vi "Actor Core.vi"(8 "error in":errorcluster, 11 "Measurement Señal Actualizable in":refnum<class "Measurement Señal Actualizable.lvclass">) -> (0 "error out":errorcluster, 3 "Actor out":refnum<class "Actor.lvclass">)   [LabVIEW 2020, in "Measurement Señal Actualizable.lvlib" / "Measurement Señal Actualizable.lvclass"]
doc: "(<B>Filename</B>: Actor Framework.lvlib:Actor.lvclass:Actor Core.vi)\n\nReceives messages to the actor, reacts to them, and initiates any error handling that may shut the actor down.\n\nDescendant classes may override this VI to append parallel tasks for the actor to complete while it handles messages. Overrides use the Call Parent Class Method node."
uses:
  C:/Program Files (x86)/National Instruments/LabVIEW 2020/vi.lib/ActorFramework/Actor/Actor.lvclass
  <vilib>/ActorFramework/Actor/Actor.lvclass
  <vilib>/ActorFramework/Actor/Actor.lvclass/Actor.ctl
  <vilib>/ActorFramework/Message Enqueuer/Message Enqueuer.lvclass/Message Enqueuer.ctl
  <vilib>/ActorFramework/Message Enqueuer/Enqueue.vi
  C:/Program Files (x86)/National Instruments/LabVIEW 2020/vi.lib/ActorFramework/Message/Message.lvclass
  <vilib>/ActorFramework/Message Priority Queue/Priority Enqueue.vi
  <vilib>/measure/NI_MABase.lvlib
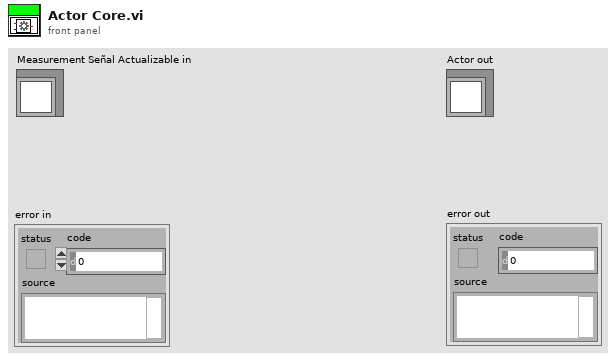
[diagram p1: front panel]
types:
  T1 = cluster{"frecuencia":dbl, "Amplitud":dbl, "Tipo de señal":enum16{"Sine Wave", "Triangle Wave", "Square Wave", "Sawtooth Wave"}}
  T2 = cluster{"Start/stop HL Event":refnum<user-event>, "Exit Event":refnum<user-event>, "Parametros Graph event":refnum<user-event>}
  T3 = enum16{"Sine Wave", "Triangle Wave", "Square Wave", "Sawtooth Wave"}
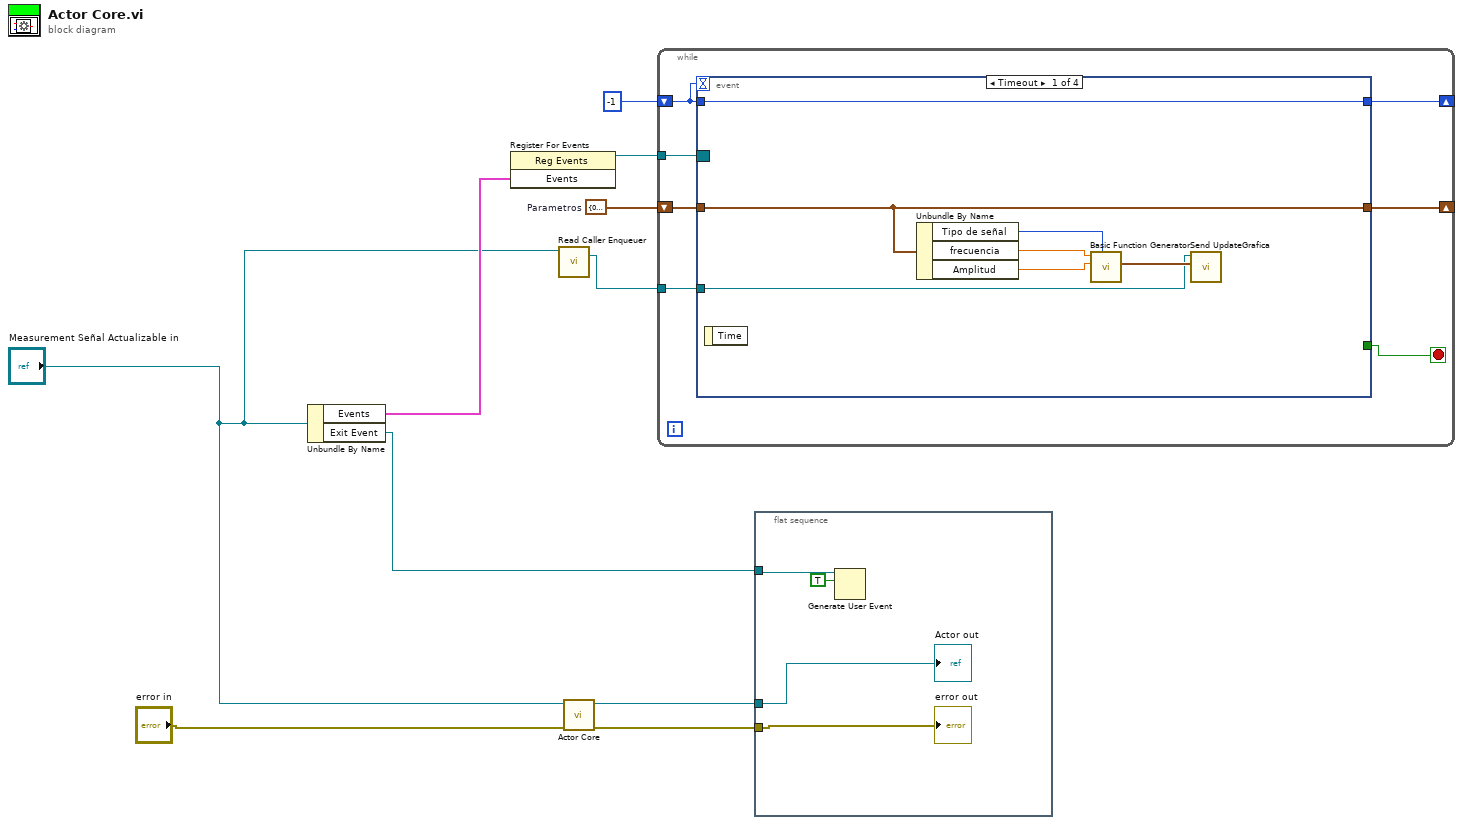
[diagram p0: block diagram]
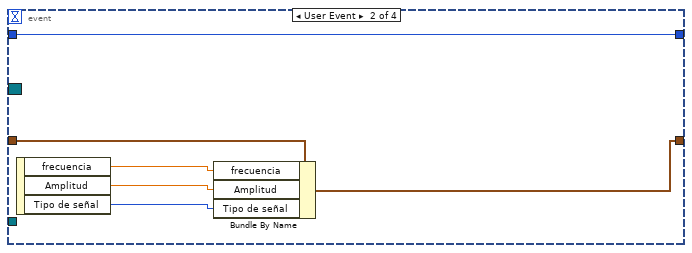
[diagram p2: hidden frame]
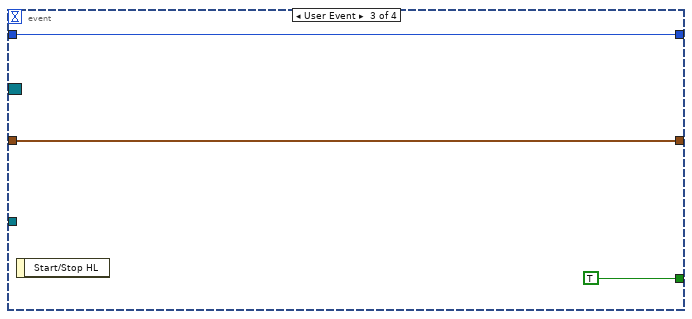
[diagram p3: hidden frame]
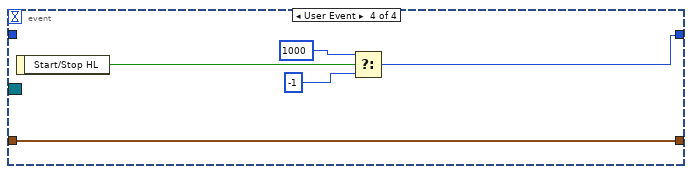
[diagram p4: hidden frame]
diagram:
  w2 = T1 {"frecuencia"=0.0, "Amplitud"=0.0, "Tipo de señal"=enum."Sine Wave"}  # Parametros
  n1 = Unbundle By Name("Measurement Señal Actualizable in") -> ("Events"=w6:T2, "Exit Event"=w7:refnum<user-event>)
  n2 = register-events(w6) -> (reference out=w4:refnum<event-registration>)  [unwired: 2 in, 1 out]
  n3 = call <vilib>:"Read Caller Enqueuer.vi"("Actor"="Measurement Señal Actualizable in") -> ("Caller Enqueuer"=w1:refnum<class "Message Enqueuer.lvclass">)  [unwired: 10 in]
  n4 = call-parent "Actor Core.vi"("error in"="error in", "Actor in"="Measurement Señal Actualizable in") -> ("error out"=w10:errorcluster, "Actor out"=w9:refnum<class "Actor.lvclass">)  [unwired: 8 in]
  n5 = while {
    tunnel: w4 -> [w17]
    shift-right: [w16] -> _
    shift-left: -1 -> [w15]
    shift-right: [w13] -> _
    shift-left: w2 -> [w14]
    tunnel: w1 -> [w12]
    stop <- w11 stop-if-true
    n6 = event shown="[0] Timeout" {
      selector: w17 -> [_ _ _ _]
      dyn-events: _ -> [_ _ _ _]
      timeout: w15 -> [_ _ _ _]
      tunnel: w15 -> [w24 w25 w33 _]
      tunnel: [w24 w25 w33 w34] -> w16
      tunnel: w14 -> [w23 w30 w32 w38]
      tunnel: [w23 w29 w32 w38] -> w13
      tunnel: w12 -> [w18 _ _ _]
      tunnel: [_ _ TRUE _] -> w11
      event Timeout {
        n7 = event-data() -> ()  [unwired: 1 in, 1 out]
        n8 = Unbundle By Name(w23) -> ("Tipo de señal"=w20:T3, "frecuencia"=w21:dbl, "Amplitud"=w22:dbl)
        n9 = call <vilib>:"Basic Function Generator.vi"("signal type"=w20, "amplitude"=w22, "frequency"=w21) -> ("signal out"=w19:waveform(dbl))  [unwired: 6 in, 2 out]
        n10 = call "Send UpdateGrafica.vi"("event data"=w19, "Message Enqueuer"=w18) -> ()  [unwired: 8 in, 2 out]
      }
      event User Event {
        n11 = event-data() -> ("frecuencia"=w28:dbl, "Amplitud"=w27:dbl, "Tipo de señal"=w26:T3)  [unwired: 1 in]
        n12 = Bundle By Name(cluster=w30, "frecuencia"=w28, "Amplitud"=w27, "Tipo de señal"=w26) -> (w29:T1)
      }
      event User Event {
        n13 = event-data() -> ()  [unwired: 1 in, 1 out]
      }
      event User Event {
        n14 = event-data() -> ("Start/Stop HL"=w37:bool)  [unwired: 1 in]
        n15 = Select(t=1000, s=w37, f=-1) -> (s? t:f=w34:i32)
      }
    }
  }
  n16 = flat-sequence {
    tunnel: w10 -> [w42]
    tunnel: w9 -> [w41]
    tunnel: w7 -> [w40]
    frame #0 {
      n17 = Generate User Event(user event=w40, event data cluster=TRUE ("event data")) -> ()  [unwired: 2 in, 2 out]
      "error out" <- w42
      "Actor out" <- w41
    }
  }
